vi "Update.vi"(8 "error in (no error)":errorcluster, 11 "StatisticsDisplay in":refnum<class "StatisticsDisplay.lvclass">) -> (0 "error out":errorcluster, 3 "StatisticsDisplay out":refnum<class "StatisticsDisplay.lvclass">)   [LabVIEW 2018, in "StatisticsDisplay.lvclass"]
uses:
  StatisticsDisplay.lvclass
  Observer/Observer.lvclass
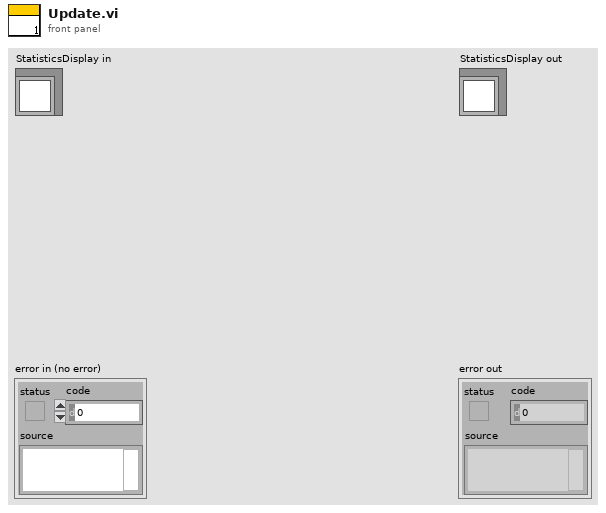
[diagram p1: front panel]
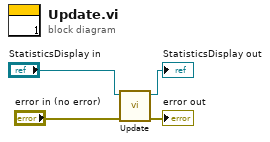
[diagram p0: block diagram]
diagram:
  n1 = call-parent "Update.vi"("error in (no error)"="error in (no error)", "Observer in"="StatisticsDisplay in") -> ("error out"=→"error out":errorcluster, "Observer out"=→"StatisticsDisplay out":refnum<class "StatisticsDisplay.lvclass">)  [unwired: 8 in]
